vi "CUST Read Configuration.vi"(10 "pseudoPdcId":i32, 11 "timeoutMs":i32) -> (3 "function return":i32)   [LabVIEW 2013, in "C37118-DLL.lvlib"]
doc: "STRONGRIDIEEEC37118DLL_API int __cdecl readConfiguration( int32_t timeoutMs, int32_t pseudoPdcId);"
uses:
  C37118-DLL.lvlib
  Auto Generated/StrongridDLL.dll
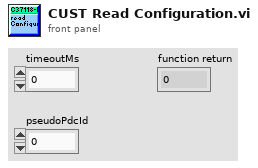
[diagram p1: front panel]
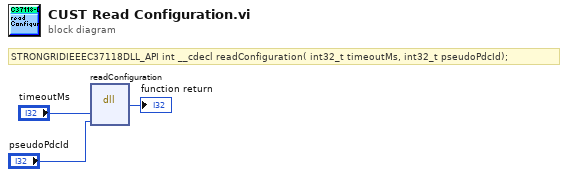
[diagram p0: block diagram]
diagram:
  # "STRONGRIDIEEEC37118DLL_API int __cdecl readConfiguration( int32_t timeoutMs, int32_t pseudoPdcId);"
  n1 = dll-call lib="C:/Prevas/Projects/statnett/AFS171 Statnett PMU Reference Library/afs171.sw/LabVIEW PRL Library LV2013/c37118-dll/labview/vi/Auto Generated/StrongridDLL.*" fn="readConfiguration"("timeoutMs"="timeoutMs", "pseudoPdcId"="pseudoPdcId") -> (→"function return":i32)  [unwired: 5 in, 2 out]
